vi "Vision Rotate Coords.vi"(8 "output cluster":cluster{"phi":dbl, "theta":dbl, "psi":dbl}, 9 "z":dbl, 10 "y":dbl, 11 "x":dbl) -> (1 "zr":dbl, 2 "yr":dbl, 3 "xr":dbl)   [LabVIEW 2016, in "Vision Drive.lvlib"]
uses:
  Vision Drive.lvlib
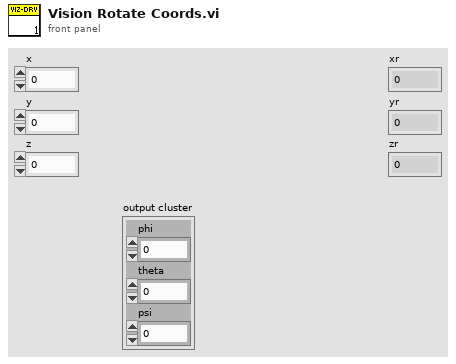
[diagram p1: front panel]
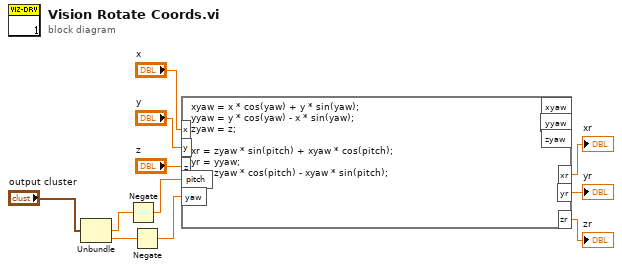
[diagram p0: block diagram]
diagram:
  n1 = Unbundle("output cluster") -> ("theta"=w4:dbl, "psi"=w3:dbl)  [unwired: 1 out]
  n2 = Negate(x=w4) -> (-x=w1:dbl)
  n3 = Negate(x=w3) -> (-x=w2:dbl)
  n4 = formula code="xyaw = x * cos(yaw) + y * sin(yaw);\nyyaw = y * cos(yaw) - x * sin(yaw);\nzyaw = z;\n\nxr = zyaw * sin(pitch) + xyaw * cos(pitch);\nyr = yyaw;\nzr = zyaw * cos(pitch) - xyaw * sin(pitch);"("x"="x", "y"="y", "z"="z", "pitch"=w1, "yaw"=w2) -> ("xr"=→"xr":dbl, "yr"=→"yr":dbl, "zr"=→"zr":dbl)  [unwired: 3 out]
